vi "Position Mini Map.vi"(8 "error in (no error)":errorcluster, 10 "VLC Window Ref":refnum<vi>, 11 "Mini Map Ref":refnum<vi>) -> (0 "error out":errorcluster)   [LabVIEW 2014]
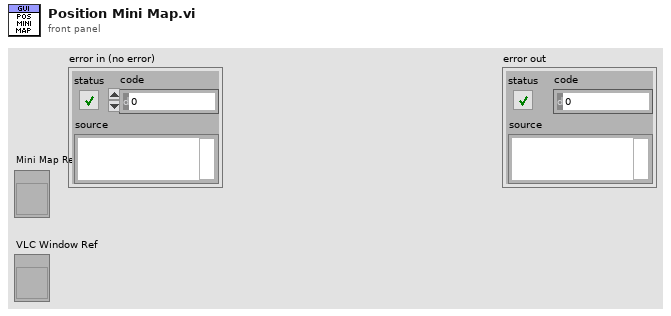
[diagram p1: front panel]
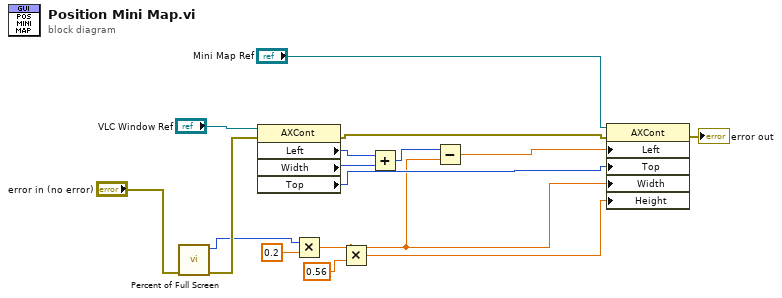
[diagram p0: block diagram]
diagram:
  n1 = call "Percent of Full Screen.vi"("error in (no error)"="error in (no error)") -> ("error out"=w11:errorcluster, "Right"=w9:i16)  [unwired: 8 in, 1 out]
  n2 = property class="AXCont"(reference="VLC Window Ref", error in=w11) -> (error out=w14:errorcluster, "Left"=w3:i32, "Width"=w2:u32, "Top"=w5:i32)  [unwired: 1 out]
  n3 = Multiply(x=w9, y=0.2) -> (x*y=w4:dbl)
  n4 = Multiply(x=w4, y=0.56) -> (x*y=w7:dbl)
  n5 = Add(x=w3, y=w2) -> (x+y=w1:u32)
  n6 = Subtract(x=w1, y=w4) -> (x-y=w6:dbl)
  n7 = property class="AXCont"(reference="Mini Map Ref", error in=w14, "Left"=w6, "Top"=w5, "Width"=w4, "Height"=w7) -> (error out=→"error out":errorcluster)  [unwired: 1 out]
